vi "WriteAttributesTest.vi"() -> ()   [LabVIEW 2013, in "examples.lvlib"]
uses:
  examples.lvlib
  vis/lv-2013/tango_vi.llb/fromStringScalar.vi
  vis/lv-2013/tango_vi.llb/fromShortScalar.vi
  vis/lv-2013/tango_vi.llb/fromLongScalar.vi
  vis/lv-2013/tango_vi.llb/fromDoubleScalar.vi
  vis/lv-2013/tango_vi.llb/tango.lvlib
panel:
  out "success":bool
  in  "value":dbl=123.456
  in  "attribute name":string="double_scalar"
  in  "value":i32=1550
  in  "attribute name":string="long_scalar"
  in  "value":i16=256
  in  "attribute name":string="short_scalar"
  in  "value":string="This is the write value..."
  in  "attribute name":string="string_scalar"
  in  "device name":string="sys/tg_test/1"
  # "TANGO  Binding for LabVIEW - Write Attributes Example"
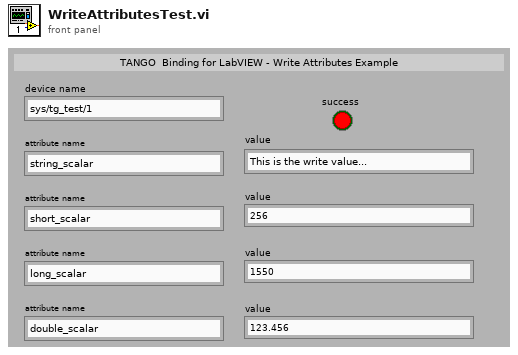
[diagram p1: front panel]
types:
  T1 = cluster{"device name":string, "attribute name":string, "quality value":i16, "quality string":string, "timestamp":dbl, "dim. x":i32, "dim. y":i32, "value":u8[], "error code":i32, "error stack":string[], "data type":u16}
  T2 = cluster{"device name":string, "attribute name":string, "quality value":i16, "quality string":string, "timestamp":dbl, "dim. x":i32, "dim. y":i32, "value":u8[], "error code":i32, "error stack":string[], "data type":u16}[]
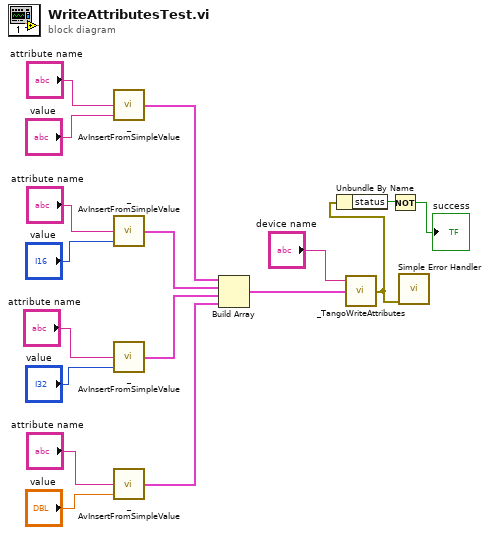
[diagram p0: block diagram]
diagram:
  n1 = call-poly "_AvInsertFromSimpleValue.vi"("value"="value", "attribute name"="attribute name") -> ("attribute value"=w13:T1)  [unwired: 1 in]
  n2 = call-poly "_AvInsertFromSimpleValue.vi"("value"="value", "attribute name"="attribute name") -> ("attribute value"=w11:T1)  [unwired: 1 in]
  n3 = call-poly "_AvInsertFromSimpleValue.vi"("value"="value", "attribute name"="attribute name") -> ("attribute value"=w8:T1)  [unwired: 1 in]
  n4 = call-poly "_AvInsertFromSimpleValue.vi"("value"="value", "attribute name"="attribute name") -> ("attribute value"=w5:T1)  [unwired: 1 in]
  n5 = Build Array(w13, w11, w8, w5) -> (w12:T2)
  n6 = call "_TangoWriteAttributes.vi"("attribute Values"=w12, "device name"="device name") -> ("error out"=w2:errorcluster)  [unwired: 1 in]
  n7 = Unbundle By Name(w2) -> ("status"=w3:bool)
  n8 = Not(x=w3) -> (.not. x?=→"success":bool)
  n9 = call <vilib>:"Simple Error Handler.vi"("error in (no error)"=w2) -> ()  [unwired: 4 in, 5 out]
